vi "Stop Core.vi"(10 "final error code":i32, 11 "Publisher in":refnum<class "Publisher.lvclass">) -> (3 "Publisher out":refnum<class "Publisher.lvclass">)   [LabVIEW 2020, in "Publisher.lvlib" / "Publisher.lvclass"]
doc: "(<B>Filename</B>: Actor Framework.lvlib:Actor.lvclass:Stop Core.vi)\n\nDefines what the actor does before it stops. Use the <B>final error code</B> input to determine whether the actor shut down in response to an error.\n\nBy default, this method does nothing. A descendant class may override it to define behavior, such as shutting down any processes the actor initiated in its override of the Actor Core method."
uses:
  Publisher.lvclass
  PPL/HDH.Actor Framework.Core.Actor.lvlibp/1abvi3w/vi.lib/ActorFramework/Message Enqueuer/Message Enqueuer.lvclass
  Publisher.lvclass/Publisher.ctl
  PPL/HDH.Actor Framework.Core.Actor.lvlibp/1abvi3w/vi.lib/ActorFramework/Actor/Actor.lvclass
  PPL/HDH.Actor Framework.Core.Actor.lvlibp/1abvi3w/vi.lib/ActorFramework/Stop Msg/Stop Msg.lvclass
  PPL/HDH.Data.Generic.lvlibp/Synchronization/Notifier/Notifier.lvclass
  PPL/HDH.Actor Framework.Core.Utility.lvlibp
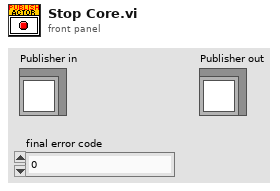
[diagram p1: front panel]
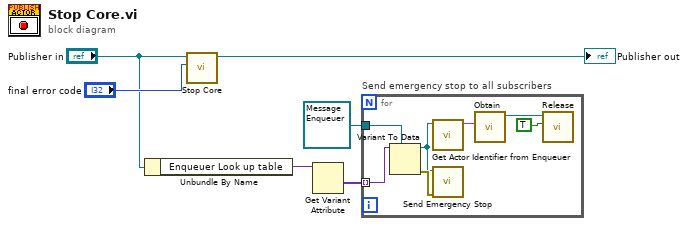
[diagram p0: block diagram]
diagram:
  n1 = Unbundle By Name("Publisher in") -> ("Enqueuer Look up table"=w3:variant)
  n2 = call-parent "Stop Core.vi"("final error code"="final error code", "Actor in"="Publisher in") -> ("Actor out"=→"Publisher out":refnum<class "Publisher.lvclass">)  [unwired: 9 in]
  n3 = Get Variant Attribute(Variant=w3) -> (values=w2:variant[])  [unwired: 3 in, 3 out]
  n4 = for "Send emergency stop to all subscribers" {
    tunnel: w2 -> [w13] mode=indexing
    tunnel: refnum<class "Message Enqueuer.lvclass"> refnum ("Subscriber Enqueuer") -> [w12]
    n5 = Variant To Data(type=w12, Variant=w13) -> (data=w10:refnum<class "Message Enqueuer.lvclass">, error out=w11:errorcluster)  [unwired: 1 in]
    n6 = call "Get Actor Identifier from Enqueuer.vi"("Message Enqueuer in"=w10) -> ("Actor ID string out"=w9:string)  [unwired: 9 in, 1 out]
    n7 = call "Send Emergency Stop.vi"("error in (no error)"=w11, "Message Enqueuer"=w10) -> ()  [unwired: 9 in, 1 out]
    n8 = call "Obtain.vi"("Name (\"\")"=w9) -> ("Notifier out"=w8:refnum<class "Notifier.lvclass">)  [unwired: 8 in, 2 out]
    n9 = call "Release.vi"("Force destroy? (F)"=TRUE, "Notifier in"=w8) -> ()  [unwired: 7 in, 3 out]
  }
